vi "Memory Game.vi"() -> ()   [LabVIEW 2019]
uses:
  TypeDefs/State.ctl
  TypeDefs/Application Data.ctl
panel:
  in  "Type the sequence shown":T1
  out "Number of colours memorised":i32
  out "Sequence to memorise":u32(colorbox)
  # "Memory Game"
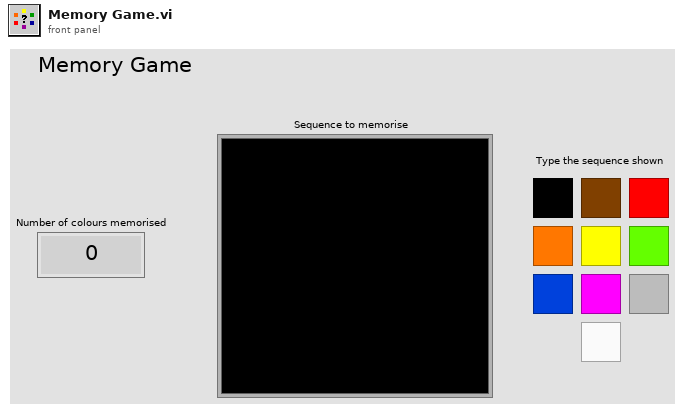
[diagram p1: front panel]
types:
  T1 = cluster{"0":bool, "7":bool, "8":bool, "9":bool, "4":bool, "5":bool, "6":bool, "1":bool, "2":bool, "3":bool}
  T2 = typedef "Application Data.ctl" = cluster{"Sequence":i32[], "Available Colours":u32[], "Wait Time (ms)":u32, "Last Key":i16, "No. Key Presses":i32, "Tally":i32}
  T3 = typedef "State.ctl" = enum16{"Initialise", "Add New Colour", "Show Sequence", "Wait For Event", "Check Key Press", "Sucess", "Failour", "Exit"}
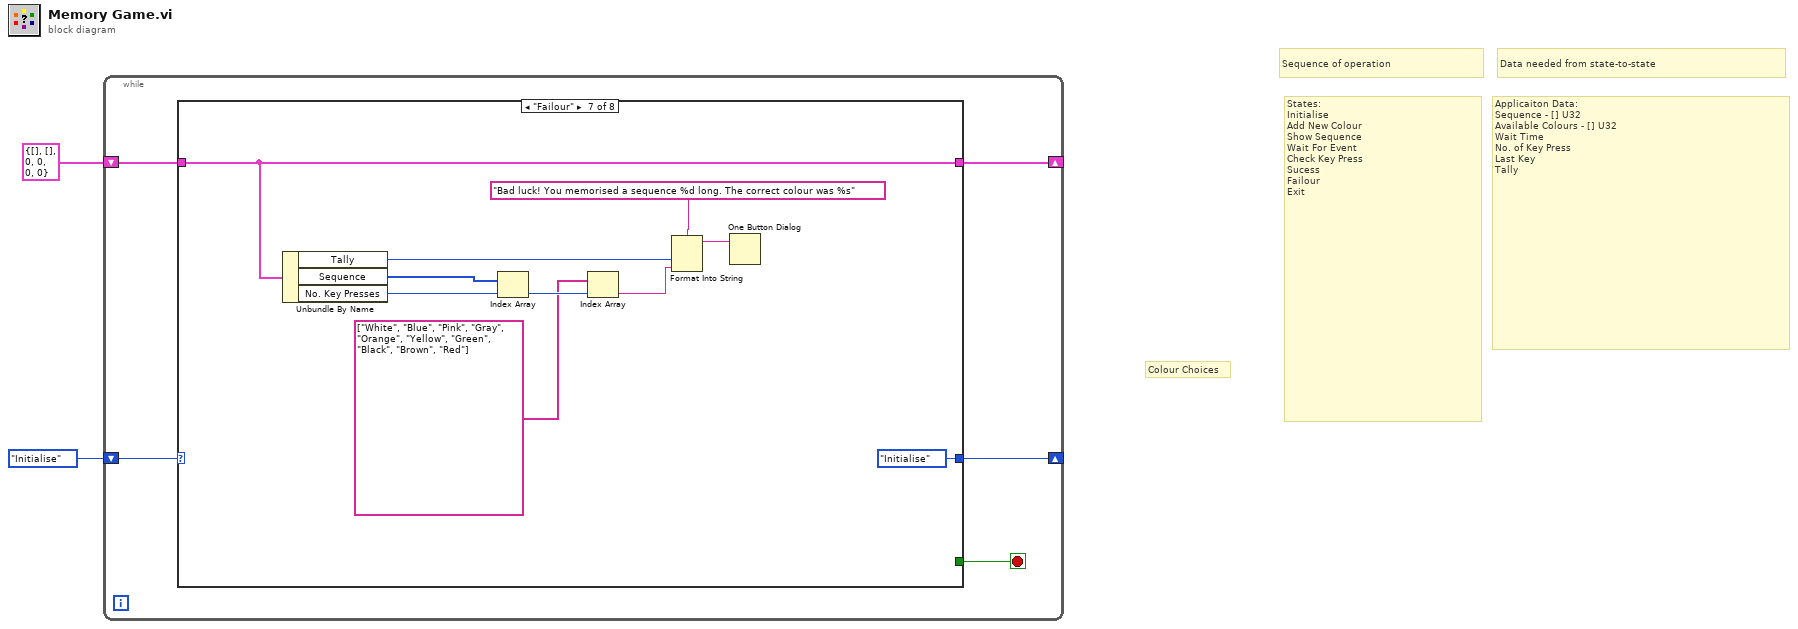
[diagram p0: block diagram]
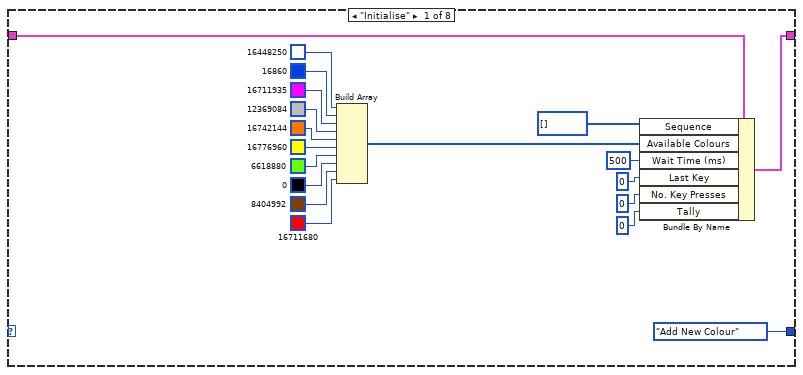
[diagram p2: hidden frame]
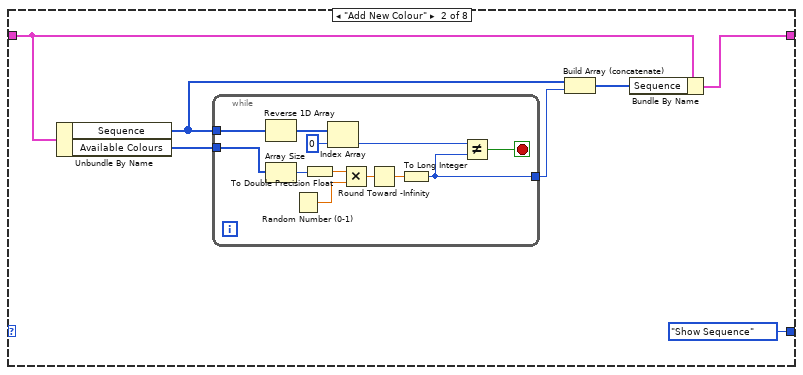
[diagram p3: hidden frame]
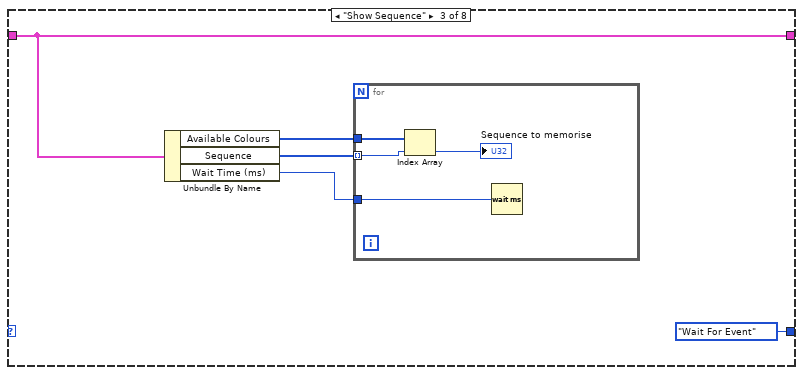
[diagram p4: hidden frame]
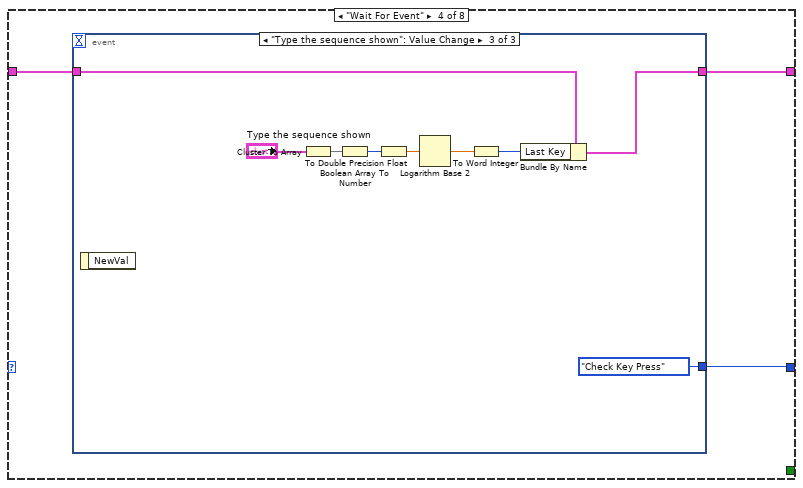
[diagram p5: hidden frame]
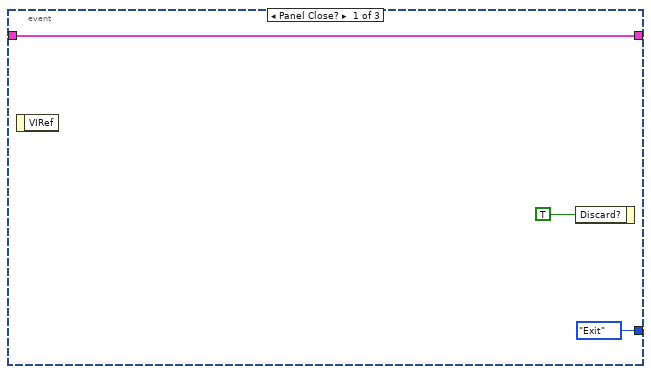
[diagram p6: hidden frame]
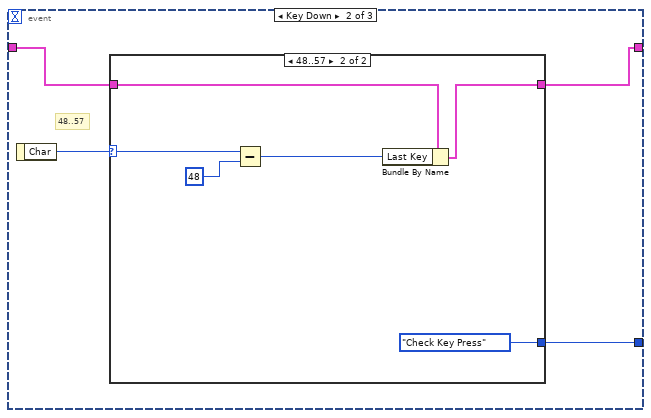
[diagram p7: hidden frame]
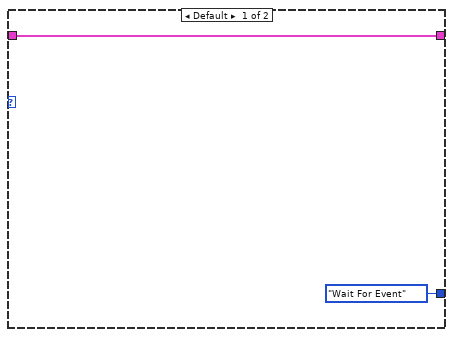
[diagram p8: hidden frame]
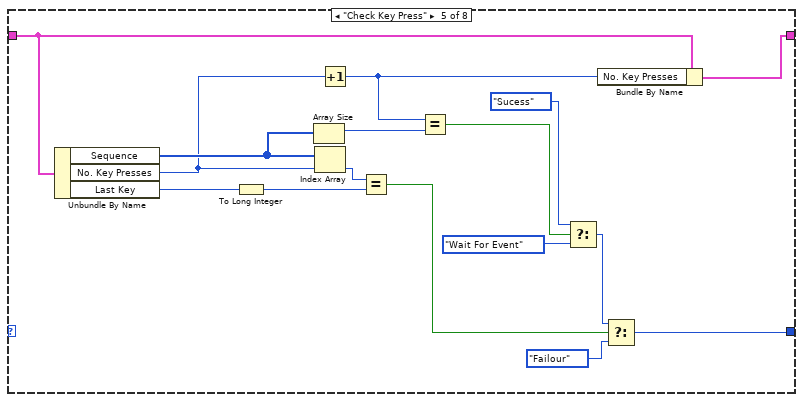
[diagram p9: hidden frame]
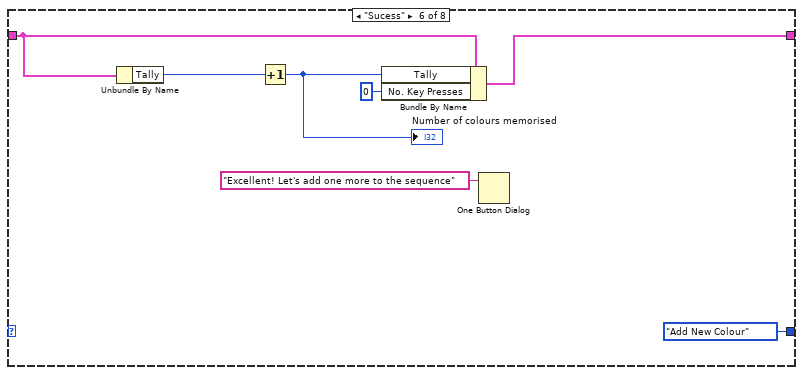
[diagram p10: hidden frame]
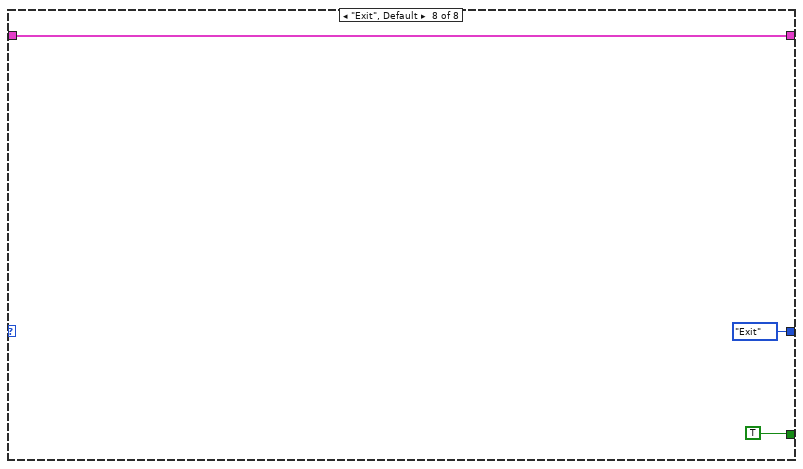
[diagram p11: hidden frame]
diagram:
  # "Data needed from state-to-state"
  # "Sequence of operation"
  # "Applicaiton Data:\nSequence - [] U32\nAvailable Colours - [] U32\nWait Time\nNo. of Key Press\nLast Key\nTally"
  # "States:\nInitialise\nAdd New Colour\nShow Sequence\nWait For Event\nCheck Key Press\nSucess\nFailour\nExit"
  # "Colour Choices"
  n1 = while {
    shift-right: [w4] -> _
    shift-left: T2 {"Sequence"=[], "Available Colours"=[], "Wait Time (ms)"=0, "Last Key"=0, "No. Key Presses"=0, "Tally"=0} -> [w5]
    shift-right: [w3] -> _
    shift-left: State."Initialise" -> [w7]
    stop <- w6 stop-if-true
    n2 = case shown="\"Failour\"" w7 {
      tunnel: [_ _ _ _ _ _ _ TRUE] -> w6
      tunnel: w5 -> [w26 w30 w50 w57 w94 w103 w112 w116]
      tunnel: [w25 w28 w50 w56 w93 w102 w112 w116] -> w4
      tunnel: [State."Add New Colour" State."Show Sequence" State."Wait For Event" w55 w91 State."Add New Colour" State."Initialise" State."Exit"] -> w3
      frame "Initialise" {
        n3 = Build Array(u32 16448250 ("Color Box"), u32 16860 ("Color Box"), u32 16711935 ("Color Box"), u32 12369084 ("Color Box"), u32 16742144 ("Color Box"), u32 16776960 ("Color Box"), u32 6618880 ("Color Box"), u32 0 ("Color Box"), u32 8404992 ("Color Box"), u32 16711680 ("Color Box")) -> (w20:u32[])
        n4 = Bundle By Name(cluster=w26, "Sequence"=i32[] [], "Available Colours"=w20, "Wait Time (ms)"=u32 500, "Last Key"=0, "No. Key Presses"=0, "Tally"=0) -> (w25:T2)
      }
      frame "Add New Colour" {
        n5 = Unbundle By Name(w30) -> ("Sequence"=w32:i32[], "Available Colours"=w33:u32[])
        n6 = while {
          tunnel: w32 -> [w45]
          tunnel: w33 -> [w42]
          tunnel: [w34] -> w31
          stop <- w35 stop-if-true
          n7 = Reverse 1D Array(array=w45) -> (reversed array=w44:i32[])
          n8 = Array Size(array=w42) -> (size(s)=w41:i32)
          n9 = Random Number (0-1)() -> (number: 0 to 1=w43:dbl)
          n10 = To Double Precision Float(number=w41) -> (double precision float=w39:dbl)
          n11 = Index Array(array=w44, index=0) -> (element=w36:i32)
          n12 = Multiply(x=w39, y=w43) -> (x*y=w40:dbl)
          n13 = Round Toward -Infinity(1:w40) -> (0:w37:dbl)
          n14 = To Long Integer(number=w37) -> (32bit integer=w34:i32)
          n15 = Not Equal?(x=w36, y=w34) -> (x != y?=w35:bool)
        }
        n16 = Build Array (concatenate)(w32, w31) -> (w29:i32[])
        n17 = Bundle By Name(cluster=w30, "Sequence"=w29) -> (w28:T2)
      }
      frame "Show Sequence" {
        n18 = Unbundle By Name(w50) -> ("Available Colours"=w48:u32[], "Sequence"=w49:i32[], "Wait Time (ms)"=w47:u32)
        n19 = for {
          tunnel: w49 -> [w53] mode=indexing
          tunnel: w48 -> [w54]
          tunnel: w47 -> [w51]
          n20 = Index Array(array=w54, index=w53) -> (element=→"Sequence to memorise":u32)
          n21 = Wait (ms)(milliseconds to wait=w51) -> ()  [unwired: 1 out]
        }
      }
      frame "Wait For Event" {
        n22 = event shown="[2] \"Type the sequence shown\": Value Change" {
          selector: _ -> [_ _ _]
          dyn-events: _ -> [_ _ _]
          timeout: _ -> [_ _ _]
          tunnel: w57 -> [w60 w63 w77]
          tunnel: [w60 w62 w75] -> w56
          tunnel: [State."Exit" w61 State."Check Key Press"] -> w55
          event Panel Close? {
            n23 = event-data() -> ()  [unwired: 1 in, 1 out]
            n24 = event-data("Discard?"=TRUE) -> ()  [unwired: 1 in, 1 out]
          }
          event Key Down {
            # "48..57"
            n25 = event-data() -> ("Char"=w64:i16)  [unwired: 1 in]
            n26 = case shown="48..57" w64 {
              selector: w64 -> [_ w70]
              tunnel: w63 -> [w66 w72]
              tunnel: [w66 w71] -> w62
              tunnel: [State."Wait For Event" State."Check Key Press"] -> w61
              frame Default {
              }
              frame 48..57 {
                n27 = Subtract(x=w70, y=i16 48) -> (x-y=w68:i16)
                n28 = Bundle By Name(cluster=w72, "Last Key"=w68) -> (w71:T2)
              }
            }
          }
          event "Type the sequence shown": Value Change {
            n29 = event-data() -> ()  [unwired: 1 in, 1 out]
            n30 = Cluster To Array(cluster="Type the sequence shown") -> (array=w80:bool[])
            n31 = Boolean Array To Number(Boolean array=w80) -> (number=w79:u32)
            n32 = To Double Precision Float(number=w79) -> (double precision float=w78:dbl)
            n33 = Logarithm Base 2(1:w78) -> (0:w76:dbl)
            n34 = To Word Integer(number=w76) -> (16bit integer=w73:i16)
            n35 = Bundle By Name(cluster=w77, "Last Key"=w73) -> (w75:T2)
          }
        }
      }
      frame "Check Key Press" {
        n36 = Unbundle By Name(w94) -> ("Sequence"=w85:i32[], "No. Key Presses"=w83:i32, "Last Key"=w96:i16)
        n37 = To Long Integer(number=w96) -> (32bit integer=w95:i32)
        n38 = Array Size(array=w85) -> (size(s)=w84:i32)
        n39 = Index Array(array=w85, index=w83) -> (element=w97:i32)
        n40 = Increment(x=w83) -> (x+1=w82:i32)
        n41 = Equal?(x=w97, y=w95) -> (x = y?=w92:bool)
        n42 = Equal?(x=w82, y=w84) -> (x = y?=w86:bool)
        n43 = Select(t=State."Sucess", s=w86, f=State."Wait For Event") -> (s? t:f=w89:T3)
        n44 = Bundle By Name(cluster=w94, "No. Key Presses"=w82) -> (w93:T2)
        n45 = Select(t=w89, s=w92, f=State."Failour") -> (s? t:f=w91:T3)
      }
      frame "Sucess" {
        n46 = Unbundle By Name(w103) -> ("Tally"=w99:i32)
        n47 = Increment(x=w99) -> (x+1=w98:i32)
        "Number of colours memorised" <- w98
        n48 = Bundle By Name(cluster=w103, "Tally"=w98, "No. Key Presses"=0) -> (w102:T2)
        n49 = One Button Dialog(message="Excellent! Let's add one more to the sequence") -> ()  [unwired: 1 in, 1 out]
      }
      frame "Failour" {
        n50 = Unbundle By Name(w112) -> ("Tally"=w111:i32, "Sequence"=w110:i32[], "No. Key Presses"=w109:i32)
        n51 = Index Array(array=w110, index=w109) -> (element=w108:i32)
        n52 = Index Array(array=string[] ["White", "Blue", "Pink", "Gray", "Orange", "Yellow", "Green", "Black", "Brown", "Red"], index=w108) -> (element=w106:string)
        n53 = Format Into String(format string="Bad luck! You memorised a sequence %d long. The correct colour was %s" ("message"), w111, w106) -> (resulting string=w113:string)  [unwired: 2 in, 1 out]
        n54 = One Button Dialog(message=w113) -> ()  [unwired: 1 in, 1 out]
      }
      frame "Exit", Default {
      }
    }
  }
